vi "Example XYGraph Markers.vi"() -> ()   [LabVIEW 2015]
uses:
  controls/MarkerOptions.ctl
  controls/GraphExt-Cmds.ctl
  controls/commands.ctl
  controls/markerType.ctl
  <vilib>/Utility/miscctls.llb/LVPoint32TypeDef.ctl
  <vilib>/ptbypt/NI_PtbyPt.lvlib
panel:
  in  "Options":T1={"Color"=16723218, "pen"={"Width"=2, "Style"=enum."Solid"}, "font"={"Font Name"="Arial", "Size"=14, "Strikeout?"=FALSE, "Italic?"=FALSE, "Underline?"=FALSE, "Outline?"=FALSE, "Shadow?"=FALSE, "Bold?"=FALSE, "FontColor"=6908265}, "caption"="Click to set a point marker"}
  out "XY Graph":cluster{dbl[], dbl[]}[](graph)
  # "Instructions:\nRun the VI, move the mouse over the graph.  \nRight click to change the marker type and see the new overlay.\nLeft click to follow instructions and place markers"
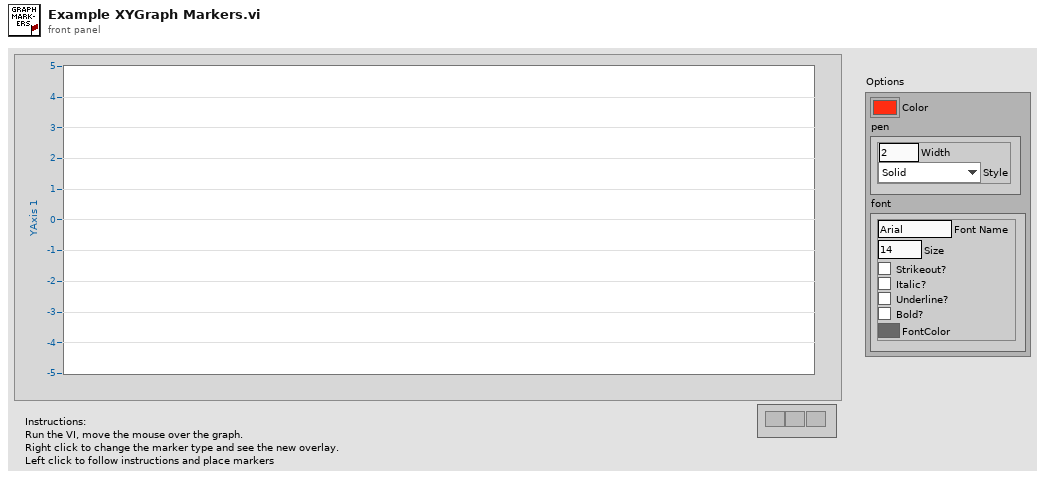
[diagram p1: front panel]
types:
  T1 = typedef "MarkerOptions.ctl" = cluster{"Color":u32, "pen":cluster{"Width":u16, "Style":enum32{"Solid", "Dash", "Dot", "DashDot", "DashDotDot"}}, "font":cluster{"Font Name":string, "Size":i16, "Strikeout?":bool, "Italic?":bool, "Underline?":bool, "Outline?":bool, "Shadow?":bool, "Bold?":bool, "FontColor":u32}, "caption":string}
  T2 = typedef "GraphExt-Cmds.ctl" = cluster{"cmd":T3, "Type":T4, "Coords":T5, "text":string}
  T3 = typedef "commands.ctl" = enum16{"up", "options", "click", "move", "type", "redraw"}
  T4 = typedef "markerType.ctl" = enum16{"point", "arrow", "horiz", "vert", "vert range", "horiz range", "box"}
  T5 = typedef "LVPoint32TypeDef.ctl" = cluster{"Horizontal":i32, "Vertical":i32}
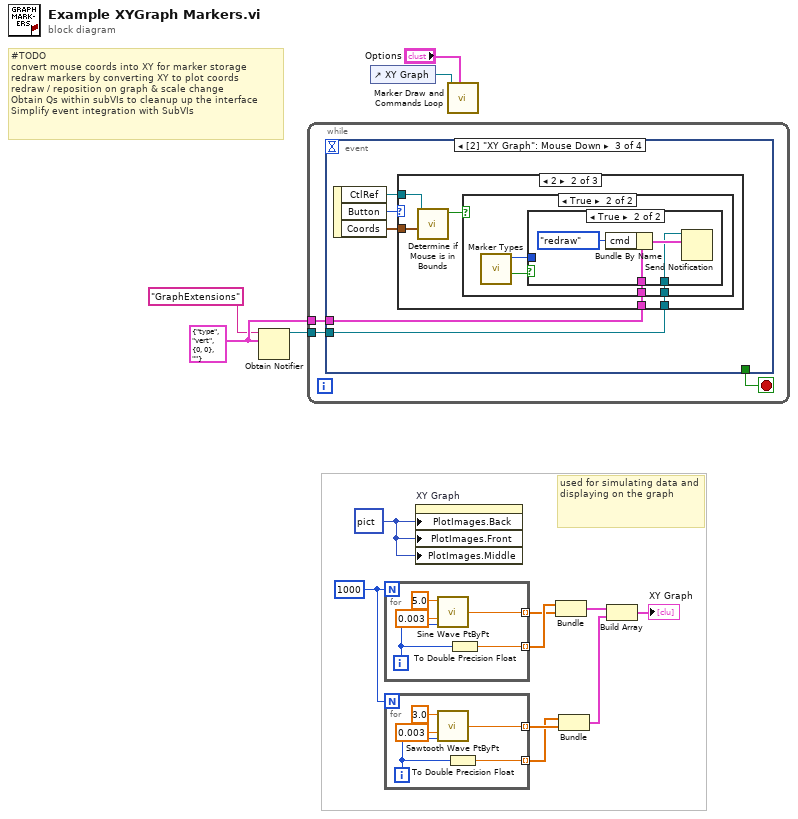
[diagram p0: block diagram]
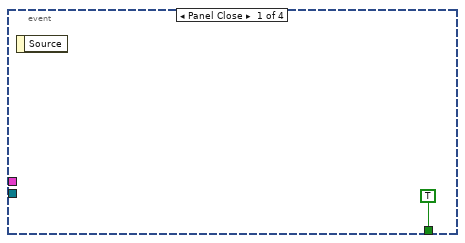
[diagram p2: hidden frame]
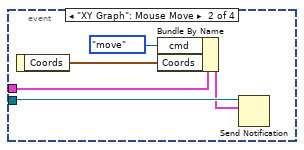
[diagram p3: hidden frame]
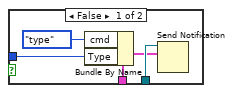
[diagram p6: hidden frame]
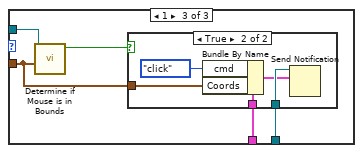
[diagram p7: hidden frame]
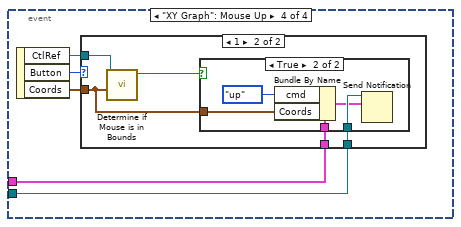
[diagram p9: hidden frame]
diagram:
  w5 = T2 {"cmd"=enum."type", "Type"=enum."vert", "Coords"={"Horizontal"=0, "Vertical"=0}, "text"=""}
  w6 = picture data[5B] ("Plot Images:Back")
  w7 = 1000
  # "used for simulating data and displaying on the graph"
  # "#TODO\nconvert mouse coords into XY for marker storage\nredraw markers by converting XY to plot coords\nredraw / reposition on graph & scale change\nObtain Qs within subVIs to cleanup up the interface\nSimplify event integration with SubVIs"
  n1 = Obtain Notifier(name (unnamed)="GraphExtensions", notification data type=w5) -> (notifier out=w4:refnum<notifier>)  [unwired: 2 in, 2 out]
  n2 = while {
    tunnel: w4 -> [w16]
    tunnel: w5 -> [w15]
    stop <- w17 stop-if-true
    n3 = event shown="[2] \"XY Graph\": Mouse Down" {
      selector: _ -> [_ _ _ _]
      dyn-events: _ -> [_ _ _ _]
      timeout: _ -> [_ _ _ _]
      tunnel: [TRUE _ _ _] -> w17
      tunnel: w16 -> [_ w23 w27 w60]
      tunnel: w15 -> [_ w22 w26 w59]
      event Panel Close {
        n4 = event-data() -> ()  [unwired: 1 in, 1 out]
      }
      event "XY Graph": Mouse Move {
        n5 = event-data() -> ("Coords"=w21:T5)  [unwired: 1 in]
        n6 = Bundle By Name(cluster=w22, "cmd"=commands."move", "Coords"=w21) -> (w20:T2)
        n7 = Send Notification(notification=w20, notifier=w23) -> ()  [unwired: 1 in, 2 out]
      }
      event "XY Graph": Mouse Down {
        n8 = event-data() -> ("CtlRef"=w24:refnum<vi>, "Button"=w28:u16, "Coords"=w25:T5)  [unwired: 1 in]
        n9 = case shown="2" w28 {
          tunnel: w27 -> [_ w33 w50]
          tunnel: w26 -> [_ w32 w51]
          tunnel: w25 -> [_ w31 w48]
          tunnel: w24 -> [_ w30 w49]
          frame Default {
          }
          frame 2 {
            n10 = call "Determine if Mouse is in Bounds.vi"("Coords"=w31, "XYGraph in"=w30) -> ("In bounds?"=w29:bool)  [unwired: 9 in]
            n11 = case shown="True" w29 {
              tunnel: w33 -> [_ w36]
              tunnel: w32 -> [_ w35]
              frame False {
              }
              frame True {
                n12 = call "Marker Types.vi"() -> ("Close"=w37:bool, "Type"=w34:T4)  [unwired: 10 in]
                n13 = case shown="True" w37 {
                  tunnel: w36 -> [w42 w43]
                  tunnel: w35 -> [w41 w44]
                  tunnel: w34 -> [w40 _]
                  frame False {
                    n14 = Bundle By Name(cluster=w41, "cmd"=commands."type", "Type"=w40) -> (w39:T2)
                    n15 = Send Notification(notification=w39, notifier=w42) -> ()  [unwired: 1 in, 2 out]
                  }
                  frame True {
                    n16 = Bundle By Name(cluster=w44, "cmd"=commands."redraw") -> (w46:T2)
                    n17 = Send Notification(notification=w46, notifier=w43) -> ()  [unwired: 1 in, 2 out]
                  }
                }
              }
            }
          }
          frame 1 {
            n18 = call "Determine if Mouse is in Bounds.vi"("Coords"=w48, "XYGraph in"=w49) -> ("In bounds?"=w47:bool)  [unwired: 9 in]
            n19 = case shown="True" w47 {
              tunnel: w51 -> [_ w56]
              tunnel: w50 -> [_ w54]
              tunnel: w48 -> [_ w52]
              frame False {
              }
              frame True {
                n20 = Bundle By Name(cluster=w56, "cmd"=commands."click", "Coords"=w52) -> (w53:T2)
                n21 = Send Notification(notification=w53, notifier=w54) -> ()  [unwired: 1 in, 2 out]
              }
            }
          }
        }
      }
      event "XY Graph": Mouse Up {
        n22 = event-data() -> ("CtlRef"=w57:refnum<vi>, "Button"=w61:u16, "Coords"=w58:T5)  [unwired: 1 in]
        n23 = case shown="1" w61 {
          tunnel: w60 -> [_ w65]
          tunnel: w59 -> [_ w66]
          tunnel: w58 -> [_ w63]
          tunnel: w57 -> [_ w64]
          frame Default {
          }
          frame 1 {
            n24 = call "Determine if Mouse is in Bounds.vi"("Coords"=w63, "XYGraph in"=w64) -> ("In bounds?"=w62:bool)  [unwired: 9 in]
            n25 = case shown="True" w62 {
              tunnel: w66 -> [_ w71]
              tunnel: w65 -> [_ w69]
              tunnel: w63 -> [_ w67]
              frame False {
              }
              frame True {
                n26 = Bundle By Name(cluster=w71, "cmd"=commands."up", "Coords"=w67) -> (w68:T2)
                n27 = Send Notification(notification=w68, notifier=w69) -> ()  [unwired: 1 in, 2 out]
              }
            }
          }
        }
      }
    }
  }
  n28 = control-ref of="XY Graph"() -> (w2:refnum<vi>)
  n29 = for {
    N: w7 -> [_]
    tunnel: [w76] -> w13 mode=indexing
    tunnel: [w72] -> w14 mode=indexing
    i -> [w75]
    n30 = call <vilib>:"Sine Wave PtByPt.vi"("time"=w75, "frequency"=0.003, "amplitude"=5.0) -> ("sine wave"=w76:dbl)  [unwired: 1 in]
    n31 = To Double Precision Float(number=w75) -> (double precision float=w72:dbl)
  }
  n32 = for {
    N: w7 -> [_]
    tunnel: [w81] -> w10 mode=indexing
    tunnel: [w77] -> w9 mode=indexing
    i -> [w80]
    n33 = call <vilib>:"Sawtooth Wave PtByPt.vi"("time"=w80, "frequency"=0.003, "amplitude"=3.0) -> ("sawtooth wave"=w81:dbl)  [unwired: 1 in]
    n34 = To Double Precision Float(number=w80) -> (double precision float=w77:dbl)
  }
  n35 = property on="XY Graph" class="XYGraph (strict)"("PlotImages.Back"=w6, "PlotImages.Front"=w6, "PlotImages.Middle"=w6) -> ()  [unwired: 2 in, 2 out]
  n36 = call "Marker Draw and Commands Loop.vi"("Options"="Options", "XY Graph"=w2) -> ()  [unwired: 10 in]
  n37 = Bundle(w14, w13) -> (w12:cluster{dbl[], dbl[]})  [unwired: 1 in]
  n38 = Bundle(w9, w10) -> (w8:cluster{dbl[], dbl[]})  [unwired: 1 in]
  n39 = Build Array(w12, w8) -> (→"XY Graph":cluster{dbl[], dbl[]}[])
